vi "hpanel_plot_hydra_counts.vi"(8 "error in (no error)":errorcluster, 10 "count_rates":T1, 11 "hydraharp_panel in":refnum<class "hydraharp_panel.lvclass">) -> (0 "error out":errorcluster, 3 "hydraharp_panel out":refnum<class "hydraharp_panel.lvclass">)   [LabVIEW 2015, in "hydraharp_panel.lvclass"]
uses:
  hydraharp_panel.lvclass
  hydraharp/hydraharp_count_rates.ctl
  UI/panel_class/panel.lvclass/panel.ctl
  hydraharp_panel.lvclass/hydraharp_panel.ctl
  UI/panel_class/panel.lvclass
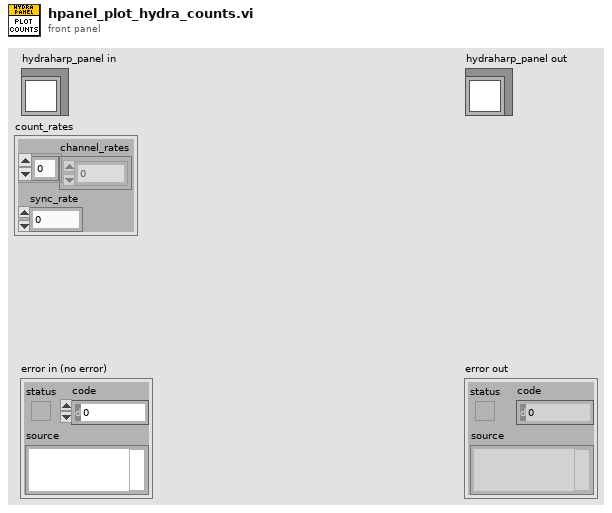
[diagram p1: front panel]
types:
  T1 = typedef "hydraharp_count_rates.ctl" = cluster{"channel_rates":i32[], "sync_rate":i32}
  T2 = typedef "ui_user_events.ctl" = cluster{"update_xy_graph":refnum<user-event>, "update_graph":refnum<user-event>, "update_chart":refnum<user-event>, "update_map":refnum<user-event>, "event_loop_stop":refnum<user-event>, "keep_map":refnum<user-event>}
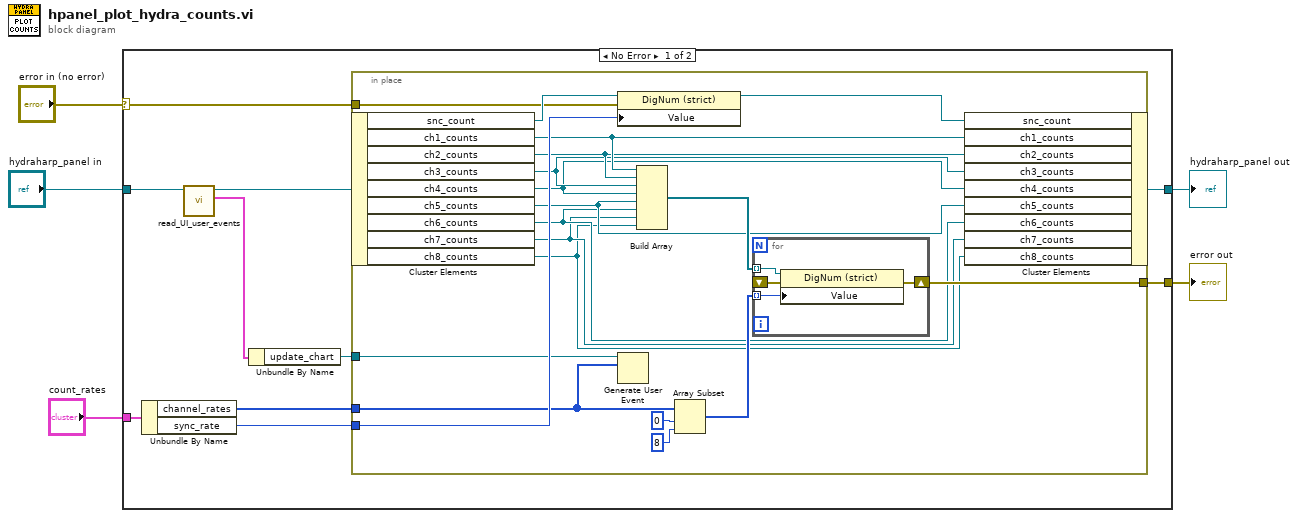
[diagram p0: block diagram]
diagram:
  n1 = case shown="No Error" "error in (no error)" {
    selector: "error in (no error)" -> [w11 w40]
    tunnel: [w10 w40] -> w4
    tunnel: [w13 w39] -> w2
    tunnel: "hydraharp_panel in" -> [w9 w39]
    tunnel: "count_rates" -> [w15 _]
    frame No Error {
      n2 = Unbundle By Name(w15) -> ("channel_rates"=w14:i32[], "sync_rate"=w12:i32)
      n3 = call "read_UI_user_events.vi"("panel in"=w9) -> ("ui_user_events"=w7:T2, "panel out"=w8:refnum<class "hydraharp_panel.lvclass">)  [unwired: 8 in, 1 out]
      n4 = Unbundle By Name(w7) -> ("update_chart"=w6:refnum<user-event>)
      n5 = in-place {
        in-place-border: w14 -> [w20]
        in-place-border: w12 -> [w31]
        in-place-border: w11 -> [w29]
        in-place-border: [w26] -> w10
        in-place-border: w6 -> [w21]
        n6 = in-place-cluster #1(w8) -> ("snc_count"=w32:refnum<vi>, "ch1_counts"=w25:refnum<vi>, "ch2_counts"=w24:refnum<vi>, "ch3_counts"=w23:refnum<vi>, "ch4_counts"=w22:refnum<vi>, "ch5_counts"=w19:refnum<vi>, "ch6_counts"=w18:refnum<vi>, "ch7_counts"=w17:refnum<vi>, "ch8_counts"=w16:refnum<vi>)
        n7 = property class="DigNum (strict)"(reference=w32, error in=w29, "Value"=w31) -> (reference out=w30:refnum<vi>)  [unwired: 1 out]
        n8 = Generate User Event(user event=w21, event data cluster=w20) -> ()  [unwired: 2 in, 2 out]
        n9 = Build Array(w25, w24, w23, w22, w19, w18, w17, w16) -> (w27:refnum<vi>[])
        n10 = Array Subset(array=w20, index=0, length=8) -> (w28:i32[])
        n11 = for {
          tunnel: w28 -> [w38] mode=indexing
          shift-right: [w35] -> w26
          shift-left: _ -> [w36]
          tunnel: w27 -> [w37] mode=indexing
          n12 = property class="DigNum (strict)"(reference=w37, error in=w36, "Value"=w38) -> (error out=w35:errorcluster)  [unwired: 1 out]
        }
        n13 = in-place-cluster #1("snc_count"=w30, "ch1_counts"=w25, "ch2_counts"=w24, "ch3_counts"=w23, "ch4_counts"=w22, "ch5_counts"=w19, "ch6_counts"=w18, "ch7_counts"=w17, "ch8_counts"=w16) -> (w13:refnum<class "hydraharp_panel.lvclass">)
      }
    }
    frame Error {
    }
  }
  "error out" <- w4
  "hydraharp_panel out" <- w2
